vi "CreateDevice.vi"(0 "Device in":refnum<class "Device.lvclass">, 5 "error in (no error)":errorcluster, 7 "FPGA API":refnum<class "FPGA API.lvclass">, 9 "ConfigInterface":refnum<class "ConfigInterface.lvclass">, 11 "SV_Publisher":refnum<class "SV_Publisher.lvclass">, 12 "Tags":T1, 13 "Logger":refnum<class "Logger.lvclass">) -> (14 "Device out":refnum<class "Device.lvclass">, 19 "error out":errorcluster)   [LabVIEW 2019, in "Device.lvclass"]
uses:
  Device.lvclass
  D:/GIT H4000/H4000/src/Proccess_class/Proccess.lvclass
  ConfigInterface_class/ConfigInterface.lvclass
  SV_Puplisher_class/SV_Publisher.lvclass
  Proccess_class/TAGs.ctl
  Logger_class/Logger.lvclass
  FPGA_API_class/FPGA API.lvclass
  MessageAMC_class/MessageAMC.lvclass
  D:/GIT H4000/H4000/src/MessageInterface_class/MessageInterface.lvclass
  Proccess_class/Proccess.lvclass/Proccess.ctl
  Device.lvclass/Device.ctl
  Proccess_class/Proccess.lvclass
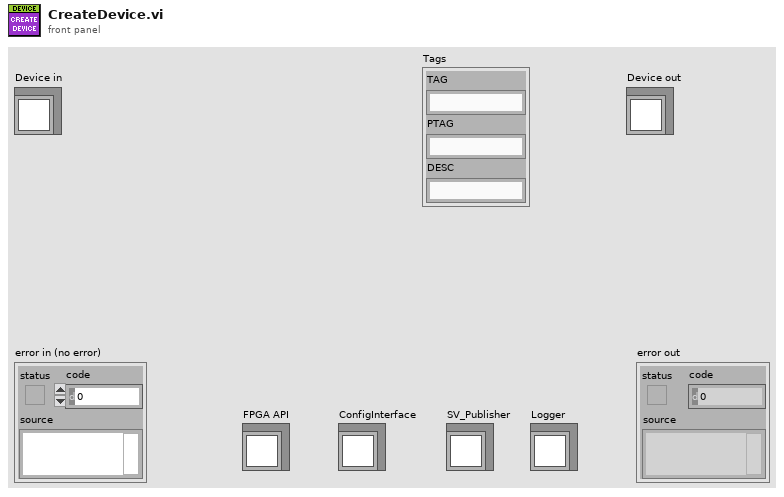
[diagram p1: front panel]
types:
  T1 = typedef "Proccess.lvclass/TAGs.ctl" = cluster{"TAG":string, "PTAG":string, "DESC":string}
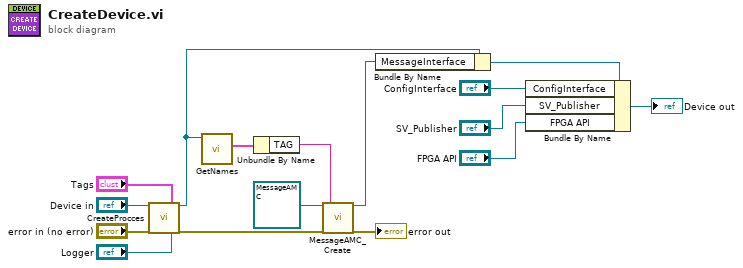
[diagram p0: block diagram]
diagram:
  n1 = call "CreateProcces.vi"("reference in"="Device in", "error in (no error)"="error in (no error)", "Tags"="Tags", "Logger"="Logger") -> ("reference out"=w2:refnum<class "Device.lvclass">, "error out"=w11:errorcluster)  [unwired: 14 in]
  n2 = call "GetNames.vi"("Proccess in"=w2) -> ("Tags"=w1:T1)  [unwired: 10 in]
  n3 = Unbundle By Name(w1) -> ("TAG"=w8:string)
  n4 = call "MessageAMC_Create.vi"("reference in"=refnum<class "MessageAMC.lvclass"> refnum ("MessageAMC"), "error in (no error)"=w11, "message queue name"=w8) -> ("amc"=w12:refnum<class "MessageAMC.lvclass">, "error out"=→"error out":errorcluster)  [unwired: 15 in]
  n5 = Bundle By Name(cluster=w2, "MessageInterface"=w12) -> (w7:refnum<class "Device.lvclass">)
  n6 = Bundle By Name(cluster=w7, "ConfigInterface"="ConfigInterface", "SV_Publisher"="SV_Publisher", "FPGA API"="FPGA API") -> (→"Device out":refnum<class "Device.lvclass">)
